vi "old version -- App - temperature sweep V0.vi"() -> ()   [LabVIEW 2010]
uses:
  state.ctl
  watch for sweep file.ctl
  save log.ctl
  save sweep table.ctl
  collect - input.ctl
  RUS/Controls/Sweep settings.ctl
  RUS/Controls/Lock-in DAQ settings.ctl
  File/Controls/Save data settings.ctl
  File/Controls/File formats.ctl
  ITC Panel.ctl
  collect.ctl
panel:
  out "Global stop indicator":bool
  in  "everything":T1(tab) caption="Tab Control"
  out "minutes/sweep":dbl=1.3333333333333333
  in  "save frequency in":bool=TRUE
  in  "Lock-in DAQ settings":T2={"Lockin mode"=enum."NI-DAQ", "DAQmx Device"="Dev2", "SR Lockin"="GPIB0::10::INSTR", "Clock Multiplier"=64, "Low-pass filter"=enum."No filtering", "Ranges and couplings "=[{"Range"=2.5, "Coupling"=10106}], "Samples per read"=10, "Record IF"=FALSE, "Auto-phase"=FALSE} {"Ranges and couplings"."Coupling" items=["default"=-1, "RSE"=10083, "NRSE"=10078, "Differential"=10106, "Pseudodifferential"=12529]}
  in  "Fast sweep settings":T3={"Update rate (Hz)"=250.0, "Start F, Hz"=900000.0, "Stop F"=1500000.0, "Number of points"=20000, "Amplitude"=2.1, "Init&amplitude"=TRUE, "IF"=1000.0, "Time constant"=0.003} {"IF" format="%#_6p"; "Amplitude" min=0.0 max=2.5; "Number of points" format="%.0p"; "Stop F" format="%#_6p"; "Start F, Hz" format="%#_6p"; "Update rate (Hz)" format="%0.2f"}
  in  "Stop RUS loop":bool
  in  "Save data settings":T4={"Save data"=TRUE, "Data Root Path"=path "C:/data/RUS/Experiment/ProbeTest/Probe10/saphire thin plate/sweep1", "File Prefix"="", "File Format"=enum."BINARY", "Save column names"=FALSE, "File Comments"="<Description of the current file>", "User/Prj"="<User Name/Project Description>"}
  in  "wait time between sweeps (min)":dbl
  in  "RUS loop":bool=TRUE
  in  "at end of every sweep":bool
  out "kHz/second":dbl=7.5
  in  "temperature boxes":T6={"LTC21 Address"="GPIB0::15::INSTR", "ITC503 Address"="GPIB0::24::INSTR", "ITC temperature"=159.22, "ITC set temperature"=159.23, "LTC temperature"=154.575, "heater"=11.7, "gas flow"=15.8, "P"=10.0, "D"=1.0, "I"=3.0, "ITC state"="X0A1C2S03H1L0\r", "nonzero temperature"=159.22}
  in  "Bypass error dialog":bool=TRUE
  out "Plot: heater/gas":cluster{dbl[], dbl[]}[](graph)
  out "heater slope, V/min":dbl=0.013240656024252648 format="%#.5f"
  out "heater average":dbl=11.680828906580725 format="%.3g"
  out "LTC T slope, K/min":dbl=0.38030539813461806 format="%#.5f"
  out "Plot: temperature":cluster{dbl[], dbl[]}[](graph)
  out "ITC Set T":dbl=159.23 format="%.3g"
  out "ITC Temperature":dbl=159.22 format="%.3g"
  out "LTC Temperature":dbl=154.575 format="%.3g"
  in  "show plot pallets":bool
  in  "set temperature to":bool
  in  "set temperature to":dbl=271.0
  in  "Tab: ITC controls":enum32{"Page 2"}(tab)
  in  "ITC panel":T7={"Locked"=FALSE, "Unlocked"=TRUE, "Remote"=FALSE, "Local"=TRUE, "in sweep"=TRUE, "start/stop sweep"=TRUE, "Sweep indicator"="IN sweep   2", "heater MANUAL"=FALSE, "heater AUTO"=TRUE, "ITC state"="X0A1C2S01H1L0\r", "gas MANUAL"=TRUE, "gas AUTO"=FALSE, "heater"=11.7, "gas flow %"=15.8} {"gas flow %" format="%.3g"; "heater" format="%.3g"}
  in  "Tab : Overheat":enum32{"Page 1"}(tab)
  in  "Over heat Temperature":dbl=350.0
  in  "Overheat protection":bool
  out "Overheat !!":bool
  in  "Tab : everything to zero":enum32{"Page 1", "Page 2"}(tab)
  in  "after (#min)":dbl=1600.0
  in  "everything to zero":bool
  in  "done":bool
  in  "to zero counter sec)":i32=132
  in  "to zero start (sec)":i32=-1
  in  "TAB: gas flow control":enum32{"Page 2"}(tab)
  in  "stop ramp up/down":bool
  in  "force ramp down now":bool
  in  "force ramp up now":bool
  in  "to":dbl=33.0
  in  "set gas flow":bool
  out "cycles between ramp up steps":i32=120
  out "ramp down in progress":bool
  out "ramp up in progress":bool
  in  "increase Gas % by":dbl=3.0
  out "(total # of ramp up steps)":i32=30
  in  "ramp up time (min)":dbl=60.0
  in  "ramp down time (min)":dbl=60.0
  in  "smallest ramp gas step":dbl=0.1
  out "(total # of ramp down steps)":i32=30
  out "ramp down steps so far":i32
  out "ramp up steps so far":i32
  out "Gas flow":dbl=15.8 format="%.2f"
  out "heater in range":bool=TRUE
  out "heater voltage":dbl=11.7 format="%.2f"
  in  "lower limit":dbl=3.0
  in  "upper limit":dbl=12.0
  in  "gas flow check interval (min)":dbl=11.0
  out "heater above":bool
  out "heater below":bool
  out "minutes since last check":i32=2
  in  "decrease Gas % by":dbl=3.0
  in  "Control Gas flow ?":bool=TRUE
  out "cycles between ramp down steps":i32=120
  in  "Tab: PID control":enum32{"Page 1"}(tab)
  in  "PID is":bool=TRUE
  out "D":dbl=1.0 format="%.2f"
  out "I":dbl=3.0 format="%.2f"
  out "P":dbl=10.0 format="%.2f"
  out "cycles since PID update":dbl=131.0 format="%.2f"
  in  "PID update every":i32=3600
  in  "PID table":dbl[][](array[numeric])=[[400.0, 10.0, 3.0, 1.0], [300.0, 10.0, 3.0, 1.0], [60.0, 10.0, 3.0, 1.0], [40.0, 10.0, 3.0, 1.0], [20.0, 30.0, 0.5, 0.2], [10.0, 40.0, 0.5, 0.2], [1.0, 50.0, 0.2, 0.2], [0.0, 50.0, 0.2, 0.2]]
  out "Uploading ...":bool
  in  "Tab : Upload Sweep table":enum32{"Page 1"}(tab)
  out "Sweep Rates , \nmin/K":dbl[][](array[numeric])=[[1.3761467889908257], [13.333333333333334], [8.0], [-0.0], [nan], [nan], [nan], [nan], [nan], [nan], [nan], [nan], [nan], [nan], [nan], [0.0]]
  out "current set \ntemperature":dbl=91.0
  in  "start \nset temperature":dbl=91.0
  in  "New Sweep Table":dbl[][](array[numeric])=[[200.0, 150.0, 0.0], [260.0, 800.0, 0.0], [310.0, 400.0, 0.0], [0.0, 0.0, 0.0], [0.0, 0.0, 0.0], [0.0, 0.0, 0.0], [0.0, 0.0, 0.0], [0.0, 0.0, 0.0], [0.0, 0.0, 0.0], [0.0, 0.0, 0.0], [0.0, 0.0, 0.0], [0.0, 0.0, 0.0], [0.0, 0.0, 0.0], [0.0, 0.0, 0.0], [0.0, 0.0, 0.0], [295.0, 0.0, 0.0]]
  in  "Read Sweep Table in the box":bool
  out "Sweep Table":dbl[][](array[numeric])=[[200.0, 150.0, 0.0], [260.0, 800.0, 0.0], [310.0, 400.0, 0.0], [0.0, 0.0, 0.0], [0.0, 0.0, 0.0], [0.0, 0.0, 0.0], [0.0, 0.0, 0.0], [0.0, 0.0, 0.0], [0.0, 0.0, 0.0], [0.0, 0.0, 0.0], [0.0, 0.0, 0.0], [0.0, 0.0, 0.0], [0.0, 0.0, 0.0], [0.0, 0.0, 0.0], [0.0, 0.0, 0.0], [295.0, 0.0, 0.0]]
  in  "upload new sweep table":bool
  out "Sweep Rates ,\nK/min":dbl[][](array[numeric])=[[0.7266666666666667], [0.075], [0.125], [-inf], [nan], [nan], [nan], [nan], [nan], [nan], [nan], [nan], [nan], [nan], [nan], [inf]]
  out "index":dbl[][](array[numeric])=[[0.0, 1200.0, 0.0], [1.0, 1200.0, 0.0], [2.0, 500.0, 0.0], [3.0, 1399.0, 0.0], [4.0, 10.0, 1399.0], [5.0, 10.0, 1399.0], [6.0, 0.0, 0.0], [7.0, 0.0, 0.0], [8.0, 0.0, 0.0], [9.0, 0.0, 0.0], [10.0, 0.0, 0.0], [11.0, 0.0, 0.0], [12.0, 0.0, 0.0], [13.0, 0.0, 0.0], [14.0, 0.0, 0.0], [15.0, 0.0, 0.0]]
  in  "New Sweep Sequence":dbl[][](array[numeric])=[[150.0, 1399.0, 0.0], [20.0, 1399.0, 0.0], [150.0, 1399.0, 0.0], [300.0, 1399.0, 0.0], [295.0, 10.0, 1399.0], [295.0, 10.0, 1399.0]]
  in  "upload new sweep sequence":bool
  in  "watch for sweep files in":T8={"file path"=path "C:/data/RUS/Experiment/ProbeTest/Probe10/saphire thin plate/sweep1", "Watch for sweep files?"=FALSE}
  out "milliseconds per cycle":u32=1000
  in  "Save sweep table":T9={"file path"=path "C:/data/RUS/Experiment/ProbeTest/probe9/LSCO_13/Sweep1", "Save sweep table?"=FALSE}
  in  "save log":T10={"file path"=path "C:/data/RUS/Experiment/ProbeTest/Probe10/saphire thin plate/sweep1", "Save log?"=TRUE, "every # of sec"=2}
  in  "bookkeeping":T11={"time(min)"=0.0, "T (ITC )"=159.22, "T (ITC, set)"=159.23, "heater"=11.7, "gas"=15.8, "T (ITC)  - T (ITC, set)"=-0.01654530309031088, "T (LTC)  - T (ITC, set)"=-4.661545303090321, "heater slope"=0.013240656024252648, "LTC slope"=0.38030539813461806, "hetaer running average"=11.680828906580725, "T (LTC)"=154.575, "T (LTC) running average"=154.57645899575306}
  out "heater":dbl=11.7 format="%.3g"
  out "gas flow %":dbl=15.8 format="%.3g"
  out "history length (min)":dbl=20.0
  out "cursor position":dbl=-1.0
  out "saving sweep table to":string
  out "saving log to":string="C:\\data\\RUS\\Experiment\\ProbeTest\\Probe10\\saphire thin plate\\sweep1\\Control_ITC_Log_120811.dat"
  out "history length (sec)":i32=1200
  out "minutes":dbl=2.183333333333333
  out "seconds":i32=131
  out "sweep files in the folder":i32=-1
  in  "error in":errorcluster
  out "error out":errorcluster
  out "log line":string="time=Dec08,2011__10:59:36\tLTC=153.75300\tITC=158.40000\t ITC_set=158.42000\t\t filename=158.40000K_900_1500_120811.dat\t"
  out "writing log to":string="C:\\data\\RUS\\Experiment\\ProbeTest\\Probe10\\saphire thin plate\\sweep1\\Stability_120811.dat"
  in  "event loop":bool
  # "cycles"
  # "Temp (K)                  P                          I                         D"
  # "the paths are copied from \"data root path\" in the first page"
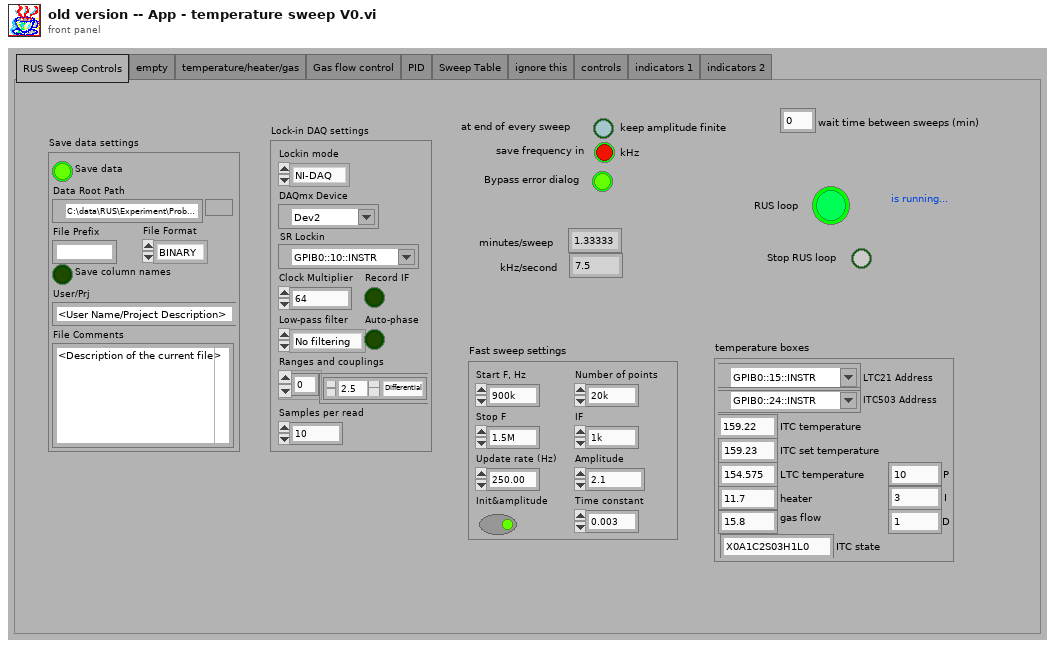
[diagram p1: front panel]
types:
  T1 = enum32{"RUS Sweep Controls", "empty", "temperature/heater/gas", "Gas flow control", "PID", "Sweep Table", "ignore this", "controls", "indicators 1", "indicators 2"}
  T2 = typedef "Lock-in DAQ settings.ctl" = cluster{"Lockin mode":enum16{"SRS", "NI-DAQ"}, "DAQmx Device":tag, "SR Lockin":refnum<visa-resource-name>, "Clock Multiplier":i32, "Low-pass filter":enum16{"No filtering", "Butterworth", "Bessel"}, "Ranges and couplings ":cluster{"Range":dbl, "Coupling":i32}[], "Samples per read":i32, "Record IF":bool, "Auto-phase":bool}
  T3 = typedef "Sweep settings.ctl" = cluster{"Update rate (Hz)":dbl, "Start F, Hz":dbl, "Stop F":dbl, "Number of points":i32, "Amplitude":dbl, "Init&amplitude":bool, "IF":dbl, "Time constant":dbl}
  T4 = typedef "Save data settings.ctl" = cluster{"Save data":bool, "Data Root Path":path, "File Prefix":string, "File Format":T5, "Save column names":bool, "File Comments":string, "User/Prj":string}
  T5 = typedef "File formats.ctl" = enum16{"TDMS", "ASCII", "BINARY"}
  T6 = typedef "state.ctl" = cluster{"LTC21 Address":refnum<visa-resource-name>, "ITC503 Address":refnum<visa-resource-name>, "ITC temperature":dbl, "ITC set temperature":dbl, "LTC temperature":dbl, "heater":dbl, "gas flow":dbl, "P":dbl, "D":dbl, "I":dbl, "ITC state":string, "nonzero temperature":dbl}
  T7 = typedef "ITC Panel.ctl" = cluster{"Locked":bool, "Unlocked":bool, "Remote":bool, "Local":bool, "in sweep":bool, "start/stop sweep":bool, "Sweep indicator":string, "heater MANUAL":bool, "heater AUTO":bool, "ITC state":string, "gas MANUAL":bool, "gas AUTO":bool, "heater":dbl, "gas flow %":dbl}
  T8 = typedef "watch for sweep file.ctl" = cluster{"file path":path, "Watch for sweep files?":bool}
  T9 = typedef "save sweep table.ctl" = cluster{"file path":path, "Save sweep table?":bool}
  T10 = typedef "save log.ctl" = cluster{"file path":path, "Save log?":bool, "every # of sec":i32}
  T11 = typedef "collect - input.ctl" = cluster{"time(min)":dbl, "T (ITC )":dbl, "T (ITC, set)":dbl, "heater":dbl, "gas":dbl, "T (ITC)  - T (ITC, set)":dbl, "T (LTC)  - T (ITC, set)":dbl, "heater slope":dbl, "LTC slope":dbl, "hetaer running average":dbl, "T (LTC)":dbl, "T (LTC) running average":dbl}
  T12 = typedef "collect.ctl" = cluster{"time(min)":dbl[], "T (ITC )":dbl[], "T (ITC, set)":dbl[], "T (LTC)":dbl[], "heater":dbl[], "gas":dbl[], "T (ITC)  - T (ITC, set)":dbl[], "T (LTC)  - T (ITC, set)":dbl[], "heater slope":dbl[], "LTC slope":dbl[], "hetaer running average":dbl[], "T (LTC) running average":dbl[]}
  T13 = enum8{"Enabled", "Disabled", "Disabled and Grayed Out"}
  T14 = enum32{"Page Enabled", "Page Disabled", "Page Disabled & Grayed"}
  T15 = cluster{"time(min)":dbl[], "T (ITC)  - T (ITC, set)":dbl[]}
  T16 = cluster{"time(min)":dbl[], "T (LTC)  - T (ITC, set)":dbl[]}
  T17 = cluster{"time(min)":dbl[], "heater slope":dbl[]}[]
  T18 = enum16{"parse", "start sweep", "stop sweep", "heater auto", "heater manual", "set heater"}
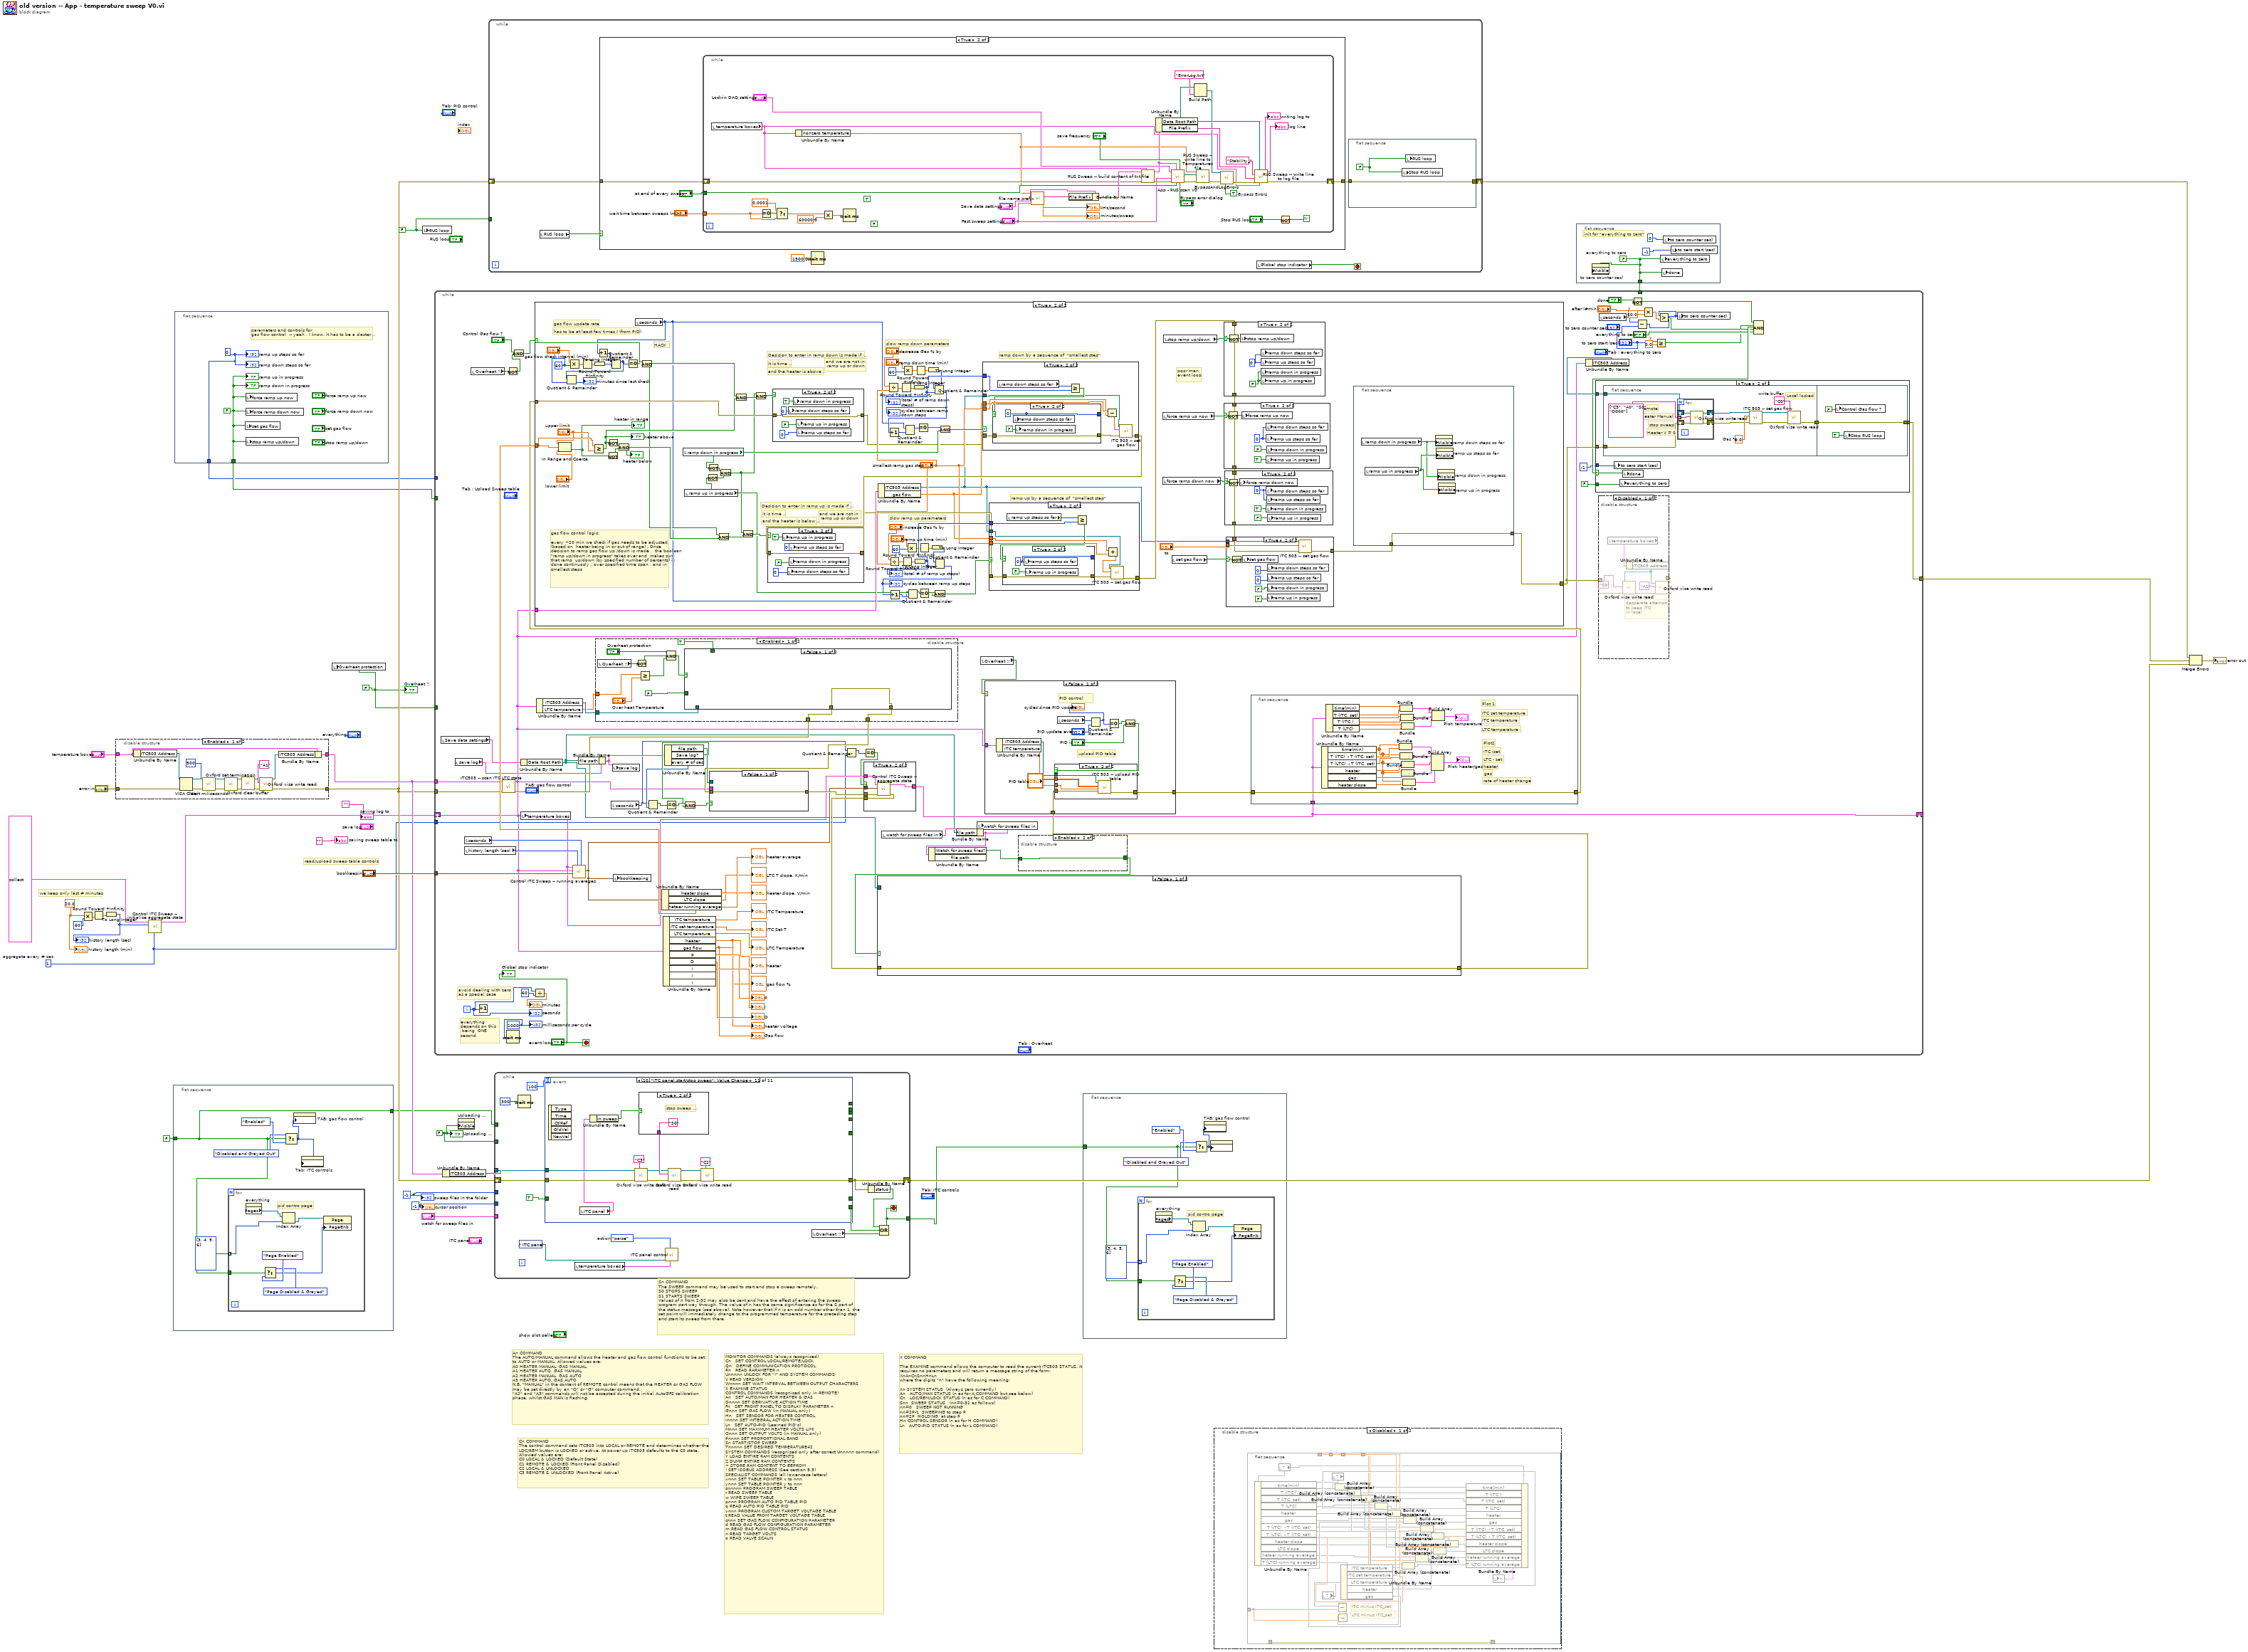
[diagram p0: block diagram]
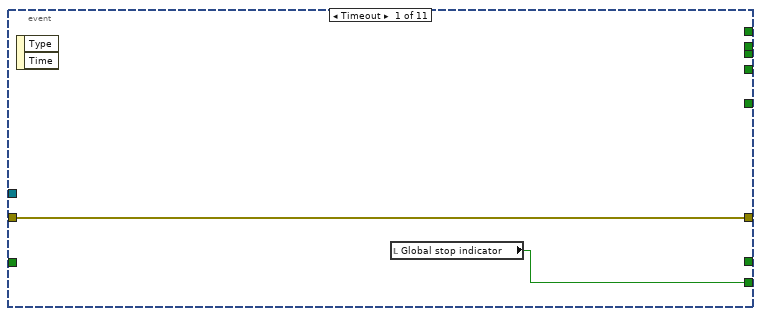
[diagram p3: hidden frame]
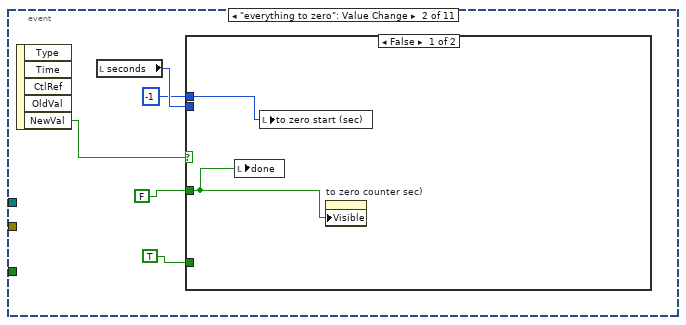
[diagram p4: hidden frame]
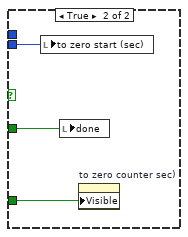
[diagram p5: hidden frame]
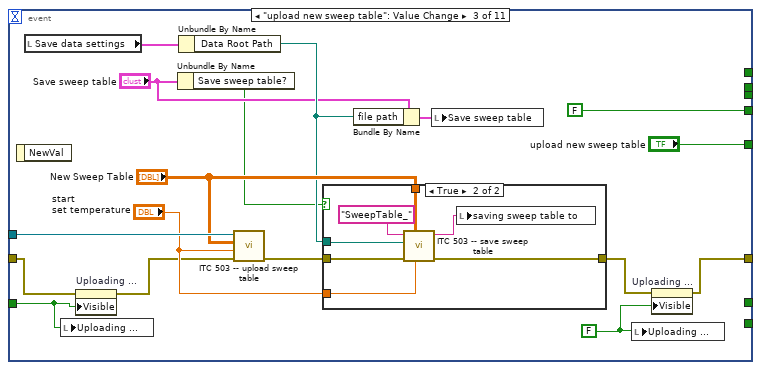
[diagram p6: hidden frame]
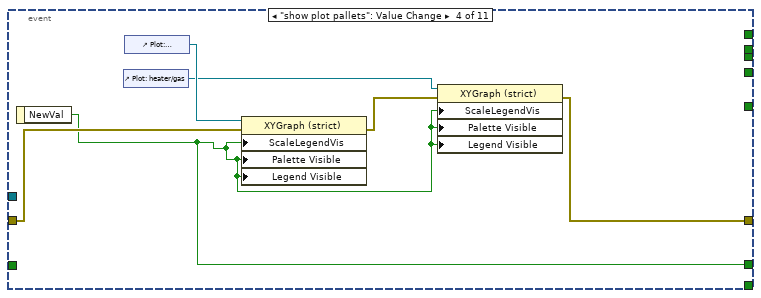
[diagram p8: hidden frame]
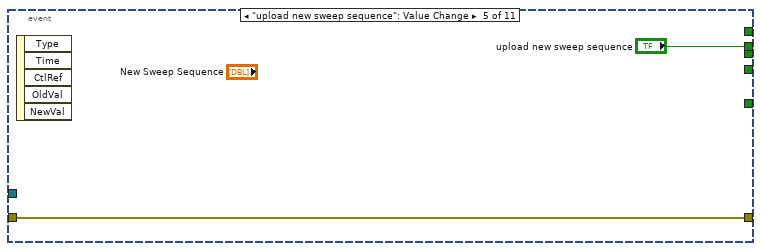
[diagram p9: hidden frame]
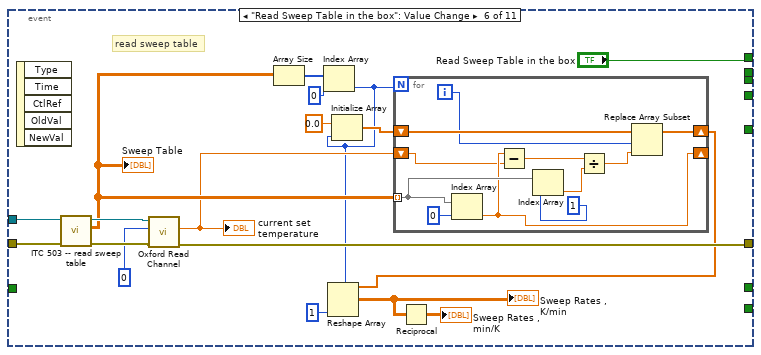
[diagram p10: hidden frame]
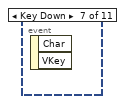
[diagram p11: hidden frame]
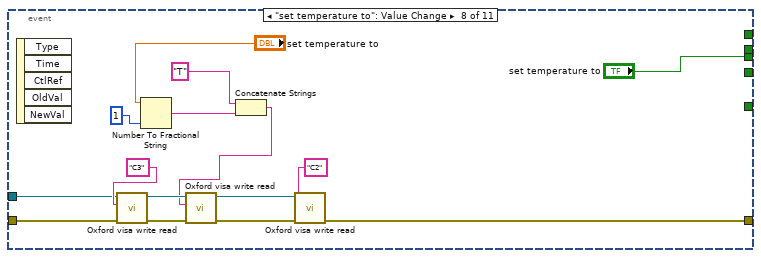
[diagram p12: hidden frame]
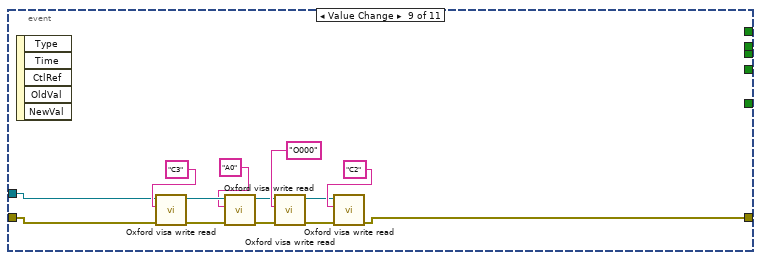
[diagram p13: hidden frame]
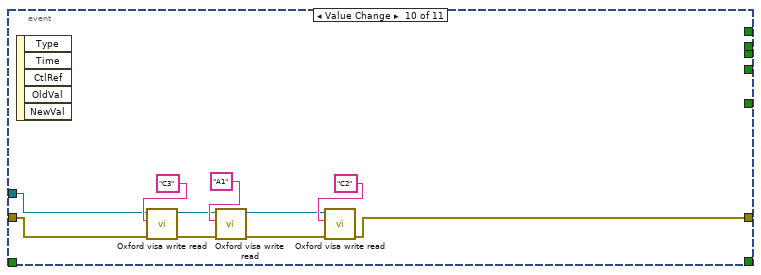
[diagram p14: hidden frame]
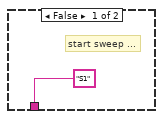
[diagram p15: hidden frame]
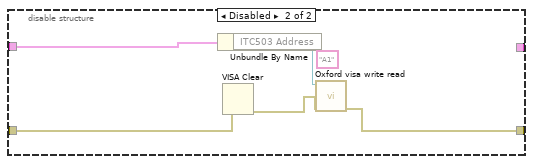
[diagram p16: hidden frame]
diagram:
  w4 = u32 1  # aggregate every # sec
  w12 = FALSE
  w11 = FALSE ("Start RUS Sweep loop")
  w14 = -1
  w29 = 20.0 ("standard deviation")
  w15 = -1 ("sweep files in the folder")
  w7 = FALSE
  # "Cn COMMAND\nThe control command sets ITC503 into LOCAL or REMOTE and determines whether the\nLOC/REM button is LOCKED or active. At power up ITC503 defaults to the C0 state.\nAllowed values are:\nC0 LOCAL & LOCKED (Default State)\nC1 REMOTE & LOCKED (Front Panel Disabled)\nC2 LOCAL & UNLOCKED\nC3 REMOTE & UNLOCKED (Front Panel Active)"
  # "An COMMAND\nThe AUTO/MANUAL command allows the heater and gas flow control functions to be set\nto AUTO or MANUAL. Allowed values are:\nA0 HEATER MANUAL, GAS MANUAL\nA1 HEATER AUTO, GAS MANUAL\nA2 HEATER MANUAL, GAS AUTO\nA3 HEATER AUTO, GAS AUTO\nN.B. \"MANUAL\" in the context of REMOTE control means that the HEATER or GAS FLOW\nmay be set directly by an \"O\" or \"G\" computer command.\n\"A2\" and \"A3\" commands will not be accepted during the initial AutoGFS calibration\nphase, whilst GAS MAN is flashing."
  # "MONITOR COMMANDS (always recognised)\nCn   SET CONTROL LOCAL/REMOTE/LOCK\nQn   DEFINE COMMUNICATION PROTOCOL\nRn   READ PARAMETER n\nUnnnnn UNLOCK FOR \"!\" AND SYSTEM COMMANDS\nV READ VERSION\nWnnnn SET WAIT INTERVAL BETWEEN OUTPUT CHARACTERS\nX EXAMINE STATUS\nCONTROL COMMANDS (recognised only in REMOTE)\nAn   SET AUTO/MAN FOR HEATER & GAS\nDnnnn SET DERIVATIVE ACTION TIME\nFn   SET FRONT PANEL TO DISPLAY PARAMETER n\nGnnn SET GAS FLOW (in MANUAL only)\nHn   SET SENSOR FOR HEATER CONTROL\nInnnn SET INTEGRAL ACTION TIME\nLn   SET AUTO-PID (Learned PID's)\nMnnn SET MAXIMUM HEATER VOLTS LIMI\nOnnn SET OUTPUT VOLTS (in MANUAL only)\nPnnnn SET PROPORTIONAL BAND\nSn START/STOP SWEEP\nTnnnnn SET DESIRED TEMPERATURE42\nSYSTEM COMMANDS (recognised only after correct Unnnnn command)\nY LOAD ENTIRE RAM CONTENTS\nZ DUMP ENTIRE RAM CONTENTS\n~ STORE RAM CONTENT TO EEPROM\n! SET ISOBUS ADDRESS (See section 8.5)\nSPECIALIST COMMANDS (all lower-case letters)\nxnnn SET TABLE POINTER x to nnn\nynnn SET TABLE POINTER y to nnn\nsnnnnn PROGRAM SWEEP TABLE\nr READ SWEEP TABLE\nw WIPE SWEEP TABLE\npnnn PROGRAM AUTO PID TABLE PID\nq READ AUTO PID TABLE PID\nvnnn PROGRAM CUSTOM TARGET VOLTAGE TABLE\nt READ VALUE FROM TARGET VOLTAGE TABLE\ncnnn SET GAS FLOW CONFIGURATION PARAMETER\nd READ GAS FLOW CONFIGURATION PARAMETER\nm READ GAS FLOW CONTROL STATUS\nn READ TARGET VOLTS\no READ VALVE SCALIN"
  # "X COMMAND\n\nThe EXAMINE command allows the computer to read the current ITC503 STATUS. It\nrequires no parameters and will return a message string of the form:\nXnAnCnSnnHnLn\nwhere the digits \"n\" have the following meaning:\n\nXn SYSTEM STATUS  (Always zero currently)\nAn   AUTO/MAN STATUS (n as for A COMMAND but see below)\nCn   LOC/REM/LOCK STATUS (n as for C COMMAND)\nSnn  SWEEP STATUS   (nn=0-32 as follows)\nnn=0   SWEEP NOT RUNNING\nnn=2P-1  SWEEPING to step P\nnn=2P  HOLDING  at step P\nHn CONTROL SENSOR (n as for H COMMAND)\nLn   AUTO-PID STATUS (n as for L COMMAND)"
  # "Sn COMMAND\nThe SWEEP command may be used to start and stop a sweep remotely.\nS0 STOPS SWEEP\nS1 STARTS SWEEP\nValues of n from 2-32 may also be sent and have the effect of entering the sweep\nprogram part way through. The value of n has the same significance as for the S part of\nthe status message (see above). Note however that if n is an odd number other than 1, the\nset point will immediately change to the programmed temperature for the preceding step\nand start its sweep from there."
  # "read/upload sweep table controls"
  # "we keep only last # minutes"
  n1 = Multiply(x=w29, y=60) -> (x*y=w32:dbl)
  n2 = Round Toward +Infinity(x=w32) -> (ceil(x): smallest int >= x=w31:dbl)
  n3 = To Long Integer(number=w31) -> (32bit integer=w21:i32)
  "history length (sec)" <- w21
  n4 = disable-structure shown="Enabled" {
    disable-tunnel: "error in" -> [w45 w53]
    disable-tunnel: [w46 w48] -> w17
    disable-tunnel: "temperature boxes" -> [w42 w51]
    disable-tunnel: [w43 _] -> w20
    frame Enabled {
      n5 = Unbundle By Name(w42) -> ("ITC503 Address"=w41:refnum<visa-resource-name>)
      n6 = VISA Clear(VISA resource name=w41, error in (no error)=w45) -> (VISA resource name out=w47:refnum<visa-resource-name>, error out=w35:errorcluster)
      n7 = call "Wait miliseconds.vi"("error in (no error)"=w35, "milliseconds to wait"=u32 500) -> ("error out"=w34:errorcluster)  [unwired: 8 in, 1 out]
      n8 = call "Oxford set termination.vi"("error in (no error)"=w34, "VISA resource name"=w47) -> ("error out"=w40:errorcluster, "VISA resource name out"=w38:refnum<visa-resource-name>)  [unwired: 8 in]
      n9 = call "Oxford clear buffer.vi"("error in (no error)"=w40, "VISA resource name"=w38) -> ("error out"=w39:errorcluster, "VISA resource name out"=w37:refnum<visa-resource-name>)  [unwired: 6 in, 2 out]
      n10 = call "Oxford visa write read.vi"("error in (no error)"=w39, "write buffer"="A1" ("Command"), "VISA resource name"=w37) -> ("error out"=w46:errorcluster, "VISA resource name out"=w36:refnum<visa-resource-name>)  [unwired: 6 in, 1 out]
      n11 = Bundle By Name(cluster=w42, "ITC503 Address"=w36) -> (w43:T6)
    }
    frame Disabled {
      (unwired) "A1" ("Command")
      n12 = Unbundle By Name(w51) -> ("ITC503 Address"=w50:refnum<visa-resource-name>)
      n13 = VISA Clear(error in (no error)=w53) -> (VISA resource name=w52:refnum<visa-resource-name>, error out=w49:errorcluster)  [unwired: 1 out]
      n14 = call "Oxford visa write read.vi"("error in (no error)"=w49, "VISA resource name"=w50) -> ("error out"=w48:errorcluster)  [unwired: 7 in, 2 out]
    }
  }
  n15 = call "Control ITC Sweep -- initialize aggregate state.vi"("time step"=w4, "length"=w21, "more state -- aggregate in"=T12 {"time(min)"=array[7200 elements], "T (ITC )"=array[7200 elements], "T (ITC, set)"=array[7200 elements], "T (LTC)"=array[7200 elements], "heater"=array[7200 elements], "gas"=array[7200 elements], "T (ITC)  - T (ITC, set)"=array[7200 elements], "T (LTC)  - T (ITC, set)"=array[7200 elements], "heater slope"=array[7200 elements], "LTC slope"=array[7200 elements], "hetaer running average"=array[7200 elements], "T (LTC) running average"=array[7200 elements]} ("thermometer snapshot -- aggregate")) -> ("more state -- aggregate out"=w6:T12)  [unwired: 7 in, 1 out]
  n16 = flat-sequence {
    tunnel: FALSE -> [w54]
    tunnel: [w54] -> w8
    frame #0 {
      n17 = for {
        tunnel: w54 -> [w63]
        tunnel: i32[] [3, 4, 5, 6] -> [w59] mode=indexing
        # "pid contro page"
        n18 = property on="everything" class="TabCtl (strict)"() -> ("Pages"=w65:refnum<vi>[])  [unwired: 2 in, 2 out]
        n19 = Select(t=T14."Page Disabled & Grayed" ("Page Enabled State"), s=w63, f=T14."Page Enabled" ("Page Enabled State")) -> (s? t:f=w60:T14)
        n20 = Index Array(array=w65, index=w59) -> (element=w64:refnum<vi>)
        n21 = property on="Property Node" class="Page"(reference=w64, "PageEnb"=w60) -> ()  [unwired: 1 in, 2 out]
      }
      n22 = Select(t=T13."Disabled and Grayed Out" ("Disabled"), s=w54, f=T13."Enabled" ("Disabled")) -> (s? t:f=w56:T13)
      n23 = property on="TAB: gas flow control" class="TabCtl (strict)"("DisabledEnum"=w56) -> ()  [unwired: 2 in, 2 out]
      n24 = property on="Tab: ITC controls" class="TabCtl (strict)"("DisabledEnum"=w56) -> ()  [unwired: 2 in, 2 out]
    }
  }
  n25 = flat-sequence {
    tunnel: [w67] -> w3
    tunnel: [w66] -> w2
    frame #0 {
      w67 = FALSE ("set gas flow manually")
      w66 = 0 ("ramp up counter")
      # "parameters and controls for \ngas flow control  -- yeah , I know, it has to be a claster .."
      n26 = local write "set gas flow"(w67) -> ()
      n27 = local write "force ramp up now"(w67) -> ()
      n28 = local write "force ramp down now"(w67) -> ()
      n29 = local write "stop ramp up/down"(w67) -> ()
      "ramp up in progress" <- w67
      "ramp down in progress" <- w67
      "ramp up steps so far" <- w66
      "ramp down steps so far" <- w66
    }
  }
  n30 = local write "Overheat protection"(w12) -> ()
  n31 = local write "RUS loop"(w11) -> ()
  n32 = while {
    tunnel: w17 -> [w118]
    tunnel: [w83] -> w23
    tunnel: w20 -> [w119]
    tunnel: "bookkeeping" -> [w116]
    tunnel: w12 -> [_]
    shift-right: [w91] -> _
    shift-left: w6 -> [w92]
    tunnel: w4 -> [w88]
    tunnel: w3 -> [_]
    tunnel: w2 -> [_]
    tunnel: w1 -> [_]
    i -> [w132]
    stop <- "event loop" stop-if-true
    w75 = 0.0  # y
    w73 = 60.0  # y
    w142 = u32 1000 ("milliseconds per cycle")
    # "everything depends on this\n being  ONE second"
    # "avoid dealing with zero \nas a special case"
    n33 = local read "Save data settings"() -> (w98:T4)
    n34 = local read "save log"() -> (w97:T10)
    n35 = local read "seconds"() -> (w115:i32)
    n36 = local read "history length (sec)"() -> (w114:i32)
    n37 = local read "Overheat !!"() -> (w102:bool)
    n38 = Increment(x=w132) -> ()  [unwired: 1 out]
    n39 = call "ITC503 -- scan ITC LTC state.vi"("error in"=w118, "state IN"=w119) -> ("error out"=w107:errorcluster, "state OUT"=w82:T6)  [unwired: 8 in]
    n40 = Wait (ms)(milliseconds to wait=w142) -> ()  [unwired: 1 out]
    n41 = Not(x=w102) -> (.not. x?=w101:bool)
    n42 = And(x="Control Gas flow ?", y=w101) -> (x .and. y?=w99:bool)
    n43 = Unbundle By Name(w98) -> ("Data Root Path"=w94:path)
    n44 = local write "temperature boxes"(w82) -> ()
    n45 = Divide(x=w132, y=60) -> (x/y=→"minutes":dbl)
    n46 = Unbundle By Name(w82) -> ("ITC503 Address"=w105:refnum<visa-resource-name>, "LTC temperature"=w104:dbl)
    n47 = call "Control ITC Sweep -- running averages.vi"("seconds"=w115, "history length (sec)"=w114, "more state"=w116, "thermometer reading"=w82, "more state -- aggregate"=w92) -> ("more state out"=w111:T11)  [unwired: 6 in]
    n48 = Bundle By Name(cluster=w97, "file path"=w94) -> (w96:T10)
    n49 = disable-structure shown="Enabled" {
      disable-tunnel: w104 -> [w368 _]
      disable-tunnel: w105 -> [w367 _]
      disable-tunnel: w107 -> [w366 w383]
      disable-tunnel: [w365 w383] -> w106
      frame Enabled {
        n50 = local read "Overheat !!"() -> (w362:bool)
        n51 = Not(x=w362) -> (.not. x?=w361:bool)
        n52 = Greater Or Equal?(x=w368, y="Over heat Temperature") -> (x >= y?=w363:bool)
        n53 = Compound Arithmetic op=AND("Overheat protection", w361, w363) -> (w364:bool)
        n54 = case shown="False" w364 {
          tunnel: w367 -> [_ w378]
          tunnel: FALSE ("Control Gas flow ?") -> [_ w375]
          tunnel: TRUE ("Boolean") -> [_ w376]
          tunnel: w366 -> [w372 w374]
          tunnel: [w372 w373] -> w365
          frame False {
          }
          frame True {
            # "Local locked"
            # "Heater V = 0"
            # "Heater Manual"
            # "Remote"
            n55 = local write "Control Gas flow ?"(w375) -> ()
            n56 = local write "Overheat !!"(w376) -> ()
            n57 = for {
              tunnel: w378 -> [w382]
              tunnel: string[] ["C3", "A0", "O0", "C0"] -> [w381] mode=indexing
              tunnel: w374 -> [w380]
              tunnel: [w379] -> w373
              n58 = call "Oxford visa write read.vi"("error in (no error)"=w380, "write buffer"=w381, "VISA resource name"=w382) -> ("error out"=w379:errorcluster)  [unwired: 6 in, 2 out]
            }
          }
        }
      }
      frame Disabled {
      }
    }
    n59 = local read "seconds"() -> (w89:i32)
    n60 = local write "save log"(w96) -> ()
    n61 = local write "bookkeeping"(w111) -> ()
    n62 = Unbundle By Name(w111) -> ("heater slope"=→"heater slope, V/min":dbl, "LTC slope"=→"LTC T slope, K/min":dbl, "hetaer running average"=w128:dbl)
    "heater average" <- w128
    n63 = case shown="True" w99 {
      selector: w99 -> [_ w267]
      tunnel: w128 -> [_ w271]
      tunnel: [w195 w270] -> w84
      tunnel: w109 -> [w195 w269]
      tunnel: w82 -> [_ w268]
      frame False {
      }
      frame True {
        w201 = 60 ("y")
        # "ramp down by a sequence of  \"smallest step\""
        # "ramp up by a sequence of  \"smallest step\""
        # "HACK"
        # "poor man \nevent loop"
        # "and we are not in\n ramp up or down"
        # "Desicion to enter in ramp up is made if ..."
        # "and the heater is below .."
        # "it is time .."
        # "and we are not in\n ramp up or down"
        # "Desicion to enter in ramp down is made if ..."
        # "and the heater is above .."
        # "it is time .."
        # "slow ramp down parameters"
        # "slow ramp up parameters"
        # "gas flow control logic: \n\nevery ~20 min we check if gas needs to be adjusted  (based on  heater being in or out of range) . Once  decision to ramp gas flow up /down is made ,  the boolean \"ramp up/down in progress\" takes over and  makes sure that ramp  up/down (by specified number of percents) is done continuosly , over specified time span , and in smallest steps"
        # "has to be at least few times I (from PID)"
        # "gas flow update rate"
        n64 = In Range and Coerce(upper limit="upper limit", x=w271, lower limit="lower limit") -> (In Range?=w262:bool)  [unwired: 1 out]
        "heater in range" <- w262
        n65 = Multiply(x="gas flow check interval (min)", y=w201) -> (x*y=w221:dbl)
        n66 = Round Toward +Infinity(x=w221) -> (ceil(x): smallest int >= x=w220:dbl)
        n67 = Greater Or Equal?(x=w271, y="upper limit") -> (x >= y?=w260:bool)
        "heater above" <- w260
        n68 = To Long Integer(number=w220) -> (32bit integer=w218:i32)
        n69 = Not(x=w262) -> (.not. x?=w264:bool)
        n70 = Not(x=w260) -> (.not. x?=w263:bool)
        n71 = And(x=w263, y=w264) -> (x .and. y?=w254:bool)
        "heater below" <- w254
        n72 = local read "seconds"() -> (w199:i32)
        n73 = Increment(x=w199) -> (x+1=w198:i32)
        n74 = Quotient & Remainder(x=w198, y=w218) -> (x-y*floor(x/y)=w202:i32)  [unwired: 1 out]
        n75 = Quotient & Remainder(x=w202, y=w201) -> (floor(x/y)=→"minutes since last check":i32)  [unwired: 1 out]
        n76 = Equal To 0?(x=w202) -> (x = 0?=w261:bool)
        n77 = And(x=w267, y=w261) -> (x .and. y?=w244:bool)
        n78 = local read "ramp down in progress"() -> (w257:bool)
        n79 = local read "ramp up in progress"() -> (w241:bool)
        n80 = Not(x=w241) -> (.not. x?=w248:bool)
        n81 = Not(x=w257) -> (.not. x?=w249:bool)
        n82 = And(x=w244, y=w254) -> (x .and. y?=w255:bool)
        n83 = And(x=w249, y=w248) -> (x .and. y?=w246:bool)
        n84 = And(x=w244, y=w260) -> (x .and. y?=w259:bool)
        n85 = And(x=w246, y=w255) -> (x .and. y?=w245:bool)
        n86 = And(x=w246, y=w259) -> (x .and. y?=w247:bool)
        n87 = case shown="True" w247 {
          tunnel: [w329 w333] -> w205
          tunnel: w269 -> [w329 w333]
          frame False {
          }
          frame True {
            n88 = local write "ramp down steps so far"(0 ("ramp down counter")) -> ()
            n89 = local write "ramp down in progress"(TRUE ("ramp down in progress")) -> ()
            n90 = local write "ramp up in progress"(FALSE ("ramp down in progress")) -> ()
            n91 = local write "ramp up steps so far"(0 ("ramp down counter")) -> ()
          }
        }
        n92 = Unbundle By Name(w268) -> ("ITC503 Address"=w196:refnum<visa-resource-name>, "gas flow"=w207:dbl)
        n93 = Divide(x="decrease Gas % by", y="smallest ramp gas step") -> (x/y=w231:dbl)
        n94 = Divide(x="increase Gas % by", y="smallest ramp gas step") -> (x/y=w236:dbl)
        n95 = Round Toward +Infinity(x=w231) -> (ceil(x): smallest int >= x=w230:dbl)
        n96 = Round Toward +Infinity(x=w236) -> (ceil(x): smallest int >= x=w234:dbl)
        n97 = Multiply(x="ramp down time (min)", y=60) -> (x*y=w217:dbl)
        n98 = Multiply(x="ramp up time (min)", y=60) -> (x*y=w212:dbl)
        n99 = To Long Integer(number=w230) -> (32bit integer=w227:i32)
        "(total # of ramp down steps)" <- w227
        n100 = To Long Integer(number=w234) -> (32bit integer=w233:i32)
        "(total # of ramp up steps)" <- w233
        n101 = Round Toward +Infinity(x=w217) -> (ceil(x): smallest int >= x=w216:dbl)
        n102 = Round Toward +Infinity(x=w212) -> (ceil(x): smallest int >= x=w211:dbl)
        n103 = To Long Integer(number=w216) -> (32bit integer=w213:i32)
        n104 = To Long Integer(number=w211) -> (32bit integer=w209:i32)
        n105 = Quotient & Remainder(x=w213, y=w227) -> (floor(x/y)=w226:i32)  [unwired: 1 out]
        "cycles between ramp down steps" <- w226
        n106 = Increment(x=w226) -> (x+1=w240:i32)
        n107 = Quotient & Remainder(x=w199, y=w240) -> (x-y*floor(x/y)=w258:i32)  [unwired: 1 out]
        n108 = Equal To 0?(x=w258) -> (x = 0?=w239:bool)
        n109 = Quotient & Remainder(x=w209, y=w233) -> (floor(x/y)=w232:i32)  [unwired: 1 out]
        "cycles between ramp up steps" <- w232
        n110 = Increment(x=w232) -> (x+1=w237:i32)
        n111 = Quotient & Remainder(x=w199, y=w237) -> (x-y*floor(x/y)=w251:i32)  [unwired: 1 out]
        n112 = Equal To 0?(x=w251) -> (x = 0?=w238:bool)
        n113 = And(x=w241, y=w238) -> (x .and. y?=w250:bool)
        n114 = And(x=w239, y=w257) -> (x .and. y?=w256:bool)
        n115 = case shown="True" w256 {
          tunnel: w207 -> [_ w345]
          tunnel: w196 -> [_ w339]
          tunnel: [w335 w338] -> w253
          tunnel: "smallest ramp gas step" -> [_ w344]
          tunnel: w227 -> [_ w341]
          tunnel: w205 -> [w335 w336]
          frame False {
          }
          frame True {
            n116 = local read "ramp down steps so far"() -> (w343:i32)
            n117 = Greater Or Equal?(x=w343, y=w341) -> (x >= y?=w342:bool)
            n118 = case shown="True" w342 {
              tunnel: [w346 w351] -> w337
              tunnel: w336 -> [w346 w351]
              tunnel: [w347 w350] -> _
              frame False {
                n119 = local read "ramp down steps so far"() -> (w347:i32)
                n120 = Increment(x=w347) -> (x+1=w348:i32)
                n121 = local write "ramp down steps so far"(w348) -> ()
              }
              frame True {
                w350 = 0 ("ramp down counter")
                n122 = local write "ramp down steps so far"(w350) -> ()
                n123 = local write "ramp down in progress"(FALSE ("ramp down in progress")) -> ()
              }
            }
            n124 = Subtract(x=w345, y=w344) -> (x-y=w340:dbl)
            n125 = call "ITC 503 -- set gas flow.vi"("error in"=w337, "Gas %"=w340, "ITC503 Address"=w339) -> ("error out"=w338:errorcluster)  [unwired: 7 in, 1 out]
          }
        }
        n126 = case shown="True" w245 {
          tunnel: w253 -> [w323 w327]
          tunnel: [w323 w327] -> w252
          frame False {
          }
          frame True {
            n127 = local write "ramp up in progress"(TRUE ("ramp up in progress")) -> ()
            n128 = local write "ramp down steps so far"(0 ("ramp down counter")) -> ()
            n129 = local write "ramp down in progress"(FALSE ("ramp down in progress")) -> ()
            n130 = local write "ramp up steps so far"(0 ("ramp up counter")) -> ()
          }
        }
        n131 = case shown="True" w250 {
          tunnel: w207 -> [_ w316]
          tunnel: w196 -> [_ w307]
          tunnel: w252 -> [w306 w314]
          tunnel: [w306 w310] -> w204
          tunnel: "smallest ramp gas step" -> [_ w315]
          tunnel: w233 -> [_ w311]
          frame False {
            # "heater above ..."
          }
          frame True {
            n132 = local read "ramp up steps so far"() -> (w313:i32)
            n133 = Greater Or Equal?(x=w313, y=w311) -> (x >= y?=w312:bool)
            n134 = case shown="True" w312 {
              tunnel: [w317 w322] -> w309
              tunnel: w314 -> [w317 w322]
              tunnel: [w318 w321] -> _
              frame False {
                n135 = local read "ramp up steps so far"() -> (w318:i32)
                n136 = Increment(x=w318) -> (x+1=w319:i32)
                n137 = local write "ramp up steps so far"(w319) -> ()
              }
              frame True {
                w321 = 0 ("ramp down counter")
                n138 = local write "ramp up steps so far"(w321) -> ()
                n139 = local write "ramp up in progress"(FALSE ("ramp down in progress")) -> ()
              }
            }
            n140 = Add(x=w316, y=w315) -> (x+y=w308:dbl)
            n141 = call "ITC 503 -- set gas flow.vi"("error in"=w309, "Gas %"=w308, "ITC503 Address"=w307) -> ("error out"=w310:errorcluster)  [unwired: 7 in, 1 out]
          }
        }
        n142 = local read "force ramp up now"() -> (w225:bool)
        n143 = local read "force ramp down now"() -> (w224:bool)
        n144 = local read "stop ramp up/down"() -> (w206:bool)
        n145 = local read "set gas flow"() -> (w242:bool)
        n146 = case shown="True" w206 {
          selector: w206 -> [_ w277]
          tunnel: w204 -> [w275 w279]
          tunnel: [w275 w279] -> w203
          frame False {
          }
          frame True {
            w280 = 0
            w278 = FALSE
            n147 = Not(x=w277) -> (.not. x?=w276:bool)
            n148 = local write "stop ramp up/down"(w276) -> ()
            n149 = local write "ramp down steps so far"(w280) -> ()
            n150 = local write "ramp up steps so far"(w280) -> ()
            n151 = local write "ramp down in progress"(w278) -> ()
            n152 = local write "ramp up in progress"(w278) -> ()
          }
        }
        n153 = case shown="True" w225 {
          selector: w225 -> [_ w291]
          tunnel: [w288 w294] -> w223
          tunnel: w203 -> [w288 w294]
          frame False {
          }
          frame True {
            w289 = 0 ("ramp up counter")
            n154 = Not(x=w291) -> (.not. x?=w292:bool)
            n155 = local write "force ramp up now"(w292) -> ()
            n156 = local write "ramp down steps so far"(w289) -> ()
            n157 = local write "ramp up steps so far"(w289) -> ()
            n158 = local write "ramp up in progress"(TRUE ("ramp up in progress")) -> ()
            n159 = local write "ramp down in progress"(FALSE) -> ()
          }
        }
        n160 = case shown="True" w224 {
          selector: w224 -> [_ w285]
          tunnel: w223 -> [w281 w287]
          tunnel: [w281 w287] -> w222
          frame False {
          }
          frame True {
            w283 = 0 ("ramp down counter")
            n161 = Not(x=w285) -> (.not. x?=w284:bool)
            n162 = local write "force ramp down now"(w284) -> ()
            n163 = local write "ramp down steps so far"(w283) -> ()
            n164 = local write "ramp down in progress"(TRUE ("ramp down in progress")) -> ()
            n165 = local write "ramp up steps so far"(w283) -> ()
            n166 = local write "ramp up in progress"(FALSE) -> ()
          }
        }
        n167 = case shown="True" w242 {
          selector: w242 -> [_ w297]
          tunnel: "to" -> [_ w302]
          tunnel: w222 -> [w295 w301]
          tunnel: [w295 w298] -> w197
          tunnel: w196 -> [_ w300]
          frame False {
          }
          frame True {
            n168 = Not(x=w297) -> (.not. x?=w296:bool)
            n169 = local write "set gas flow"(w296) -> ()
            n170 = local write "ramp down steps so far"(0 ("ramp down counter")) -> ()
            n171 = local write "ramp up steps so far"(0 ("ramp up counter")) -> ()
            n172 = local write "ramp down in progress"(FALSE ("ramp down in progress")) -> ()
            n173 = local write "ramp up in progress"(FALSE ("ramp up in progress")) -> ()
            n174 = call "ITC 503 -- set gas flow.vi"("error in"=w301, "Gas %"=w302, "ITC503 Address"=w300) -> ("error out"=w298:errorcluster)  [unwired: 7 in, 1 out]
          }
        }
        n175 = flat-sequence {
          tunnel: [w274] -> w270
          tunnel: w197 -> [w274]
          frame #0 {
            n176 = local read "ramp down in progress"() -> (w272:bool)
            n177 = local read "ramp up in progress"() -> (w273:bool)
            n178 = property on="ramp down steps so far" class="DigNum (strict)"("Visible"=w272) -> ()  [unwired: 2 in, 2 out]
            n179 = property on="ramp up steps so far" class="DigNum (strict)"("Visible"=w273) -> ()  [unwired: 2 in, 2 out]
            n180 = property on="ramp down in progress" class="Bool (strict)"("Visible"=w272) -> ()  [unwired: 2 in, 2 out]
            n181 = property on="ramp up in progress" class="Bool (strict)"("Visible"=w273) -> ()  [unwired: 2 in, 2 out]
          }
        }
      }
    }
    n182 = Unbundle By Name(w82) -> ("ITC temperature"=→"ITC Temperature":dbl, "ITC set temperature"=→"ITC Set T":dbl, "LTC temperature"=→"LTC Temperature":dbl, "heater"=→"heater voltage" →"heater":dbl, "gas flow"=→"Gas flow" →"gas flow %":dbl, "P"=→"P":dbl, "D"=→"D":dbl, "I"=→"I":dbl)  [unwired: 2 out]
    n183 = Unbundle By Name(w96) -> ("file path"=w122:path, "Save log?"=w121:bool, "every # of sec"=w120:i32)
    n184 = Quotient & Remainder(x=w89, y=w120) -> (x-y*floor(x/y)=w125:i32)  [unwired: 1 out]
    n185 = Equal To 0?(x=w125) -> (x = 0?=w124:bool)
    n186 = And(x=w124, y=w121) -> (x .and. y?=w123:bool)
    n187 = case shown="False" w123 {
      tunnel: w122 -> [_ w388]
      tunnel: [w384 w385] -> w117
      tunnel: w106 -> [w384 w386]
      tunnel: w82 -> [_ w387]
      frame False {
      }
      frame True {
        n188 = call "A - write log line.vi"("error in"=w386, "temperature boxes"=w387, "Basename"="Control_ITC_Log_" ("string"), "Base Path"=w388) -> ("error out"=w385:errorcluster, "saving log to"=w390:string)  [unwired: 6 in]
        n189 = local write "saving log to"(w390) -> ()
      }
    }
    n190 = Quotient & Remainder(x=w89, y=w88) -> (x-y*floor(x/y)=w90:u32)  [unwired: 1 out]
    n191 = Equal To 0?(x=w90) -> (x = 0?=w87:bool)
    n192 = case shown="True" w87 {
      tunnel: w117 -> [w169 w175]
      tunnel: w111 -> [_ w174]
      tunnel: [w169 w173] -> w110
      tunnel: w92 -> [w170 w172]
      tunnel: [w170 w171] -> w91
      frame False {
      }
      frame True {
        n193 = call "Control ITC Sweep -- aggregate state.vi"("error in"=w175, "more state"=w174, "more state -- aggregate in"=w172) -> ("error out"=w173:errorcluster, "more state -- aggregate out"=w171:T12)  [unwired: 7 in]
      }
    }
    n194 = local read "watch for sweep files in"() -> (w95:T8)
    n195 = Bundle By Name(cluster=w95, "file path"=w94) -> (w93:T8)
    n196 = Unbundle By Name(w93) -> ("Watch for sweep files?"=w130:bool)  [unwired: 1 out]
    n197 = local write "watch for sweep files in"(w93) -> ()
    n198 = local read "Overheat !!"() -> (w103:bool)
    n199 = disable-structure shown="Enabled" {
      disable-tunnel: w130 -> [w414 w419]
      disable-tunnel: [w413 w419] -> w129
      frame Disabled {
        # "check folder every ..."
        n200 = local read "seconds"() -> (w415:i32)
        n201 = Quotient & Remainder(x=w415, y=2) -> (x-y*floor(x/y)=w417:i32)  [unwired: 1 out]
        n202 = Equal To 0?(x=w417) -> (x = 0?=w416:bool)
        n203 = And(x=w414, y=w416) -> (x .and. y?=w413:bool)
      }
      frame Enabled {
      }
    }
    n204 = case shown="False" w129 {
      tunnel: w94 -> [_ w431]
      tunnel: w110 -> [w420 w421]
      tunnel: [w420 w421] -> w108
      frame False {
      }
      frame True {
        w430 = 60.0 ("y")
        # "hack"
        # "watch for new RUS file in sweep folder  and replace cursor every time sweep starts"
        # "date"
        n205 = Get Date/Time In Seconds() -> (seconds since 1Jan1904=w440:timestamp)
        n206 = Format Date/Time String(time format string (%c)="%m%d%y", seconds (now)=w440) -> (date/time string=w436:string)  [unwired: 1 in]
        n207 = Format Date/Time String(time format string (%c)="%B_%Y", seconds (now)=w440) -> (date/time string=w442:string)  [unwired: 1 in]
        n208 = Concatenate Strings(w442, "\\" ("time format string (%c)"), w436) -> (w443:string)
        n209 = Build Path(base path=w431, name or relative path=w443) -> (appended path=w433:path)
        n210 = Concatenate Strings("*" ("time format string (%c)"), w436, ".txt" ("time format string (%c)")) -> (w434:string)
        n211 = Path To String(path=w433) -> ()  [unwired: 1 out]
        n212 = call <vilib>:"Check if File or Folder Exists.vi"("path"=w433) -> ("file or folder exists?"=w423:bool, "dup path"=w432:path)  [unwired: 8 in, 1 out]
        n213 = local read "cursor position"() -> (w427:dbl)
        n214 = Multiply(x=w427, y=w430) -> (x*y=w428:dbl)
        n215 = Greater Or Equal To 0?(x=w427) -> (x >= 0?=w425:bool)
        n216 = Decrement(x=w428) -> (x-1=w429:dbl)
        n217 = Divide(x=w429, y=w430) -> (x/y=w426:dbl)
        n218 = And(x=w423, y=w425) -> (x .and. y?=w424:bool)
        n219 = Select(t=w426, s=w424, f=w427) -> (s? t:f=w422:dbl)
        n220 = local write "cursor position"(w422) -> ()
        n221 = property on="Plot: heater/gas" class="XYGraph (strict)"("Cursor.Cursor X"=w422) -> ()  [unwired: 2 in, 2 out]
        n222 = case shown="True" w423 {
          tunnel: w434 -> [_ w454]
          tunnel: w432 -> [_ w452]
          frame False {
            n223 = local read "watch for sweep files in"() -> (w446:T8)
            n224 = Bundle By Name(cluster=w446, "Watch for sweep files?"=FALSE) -> (w444:T8)
            n225 = local write "watch for sweep files in"(w444) -> ()
          }
          frame True {
            n226 = local read "sweep files in the folder"() -> (w449:i32)
            n227 = Less Than 0?(x=w449) -> (x < 0?=w448:bool)
            n228 = List Folder(path=w452, pattern=w454) -> (filenames=w453:string[])  [unwired: 2 in, 3 out]
            n229 = Array Size(array=w453) -> (size(s)=w451:i32)
            n230 = case shown="True" w448 {
              tunnel: w451 -> [_ w459]
              tunnel: [w458 w459] -> w450
              frame False {
                n231 = local read "sweep files in the folder"() -> (w458:i32)
              }
              frame True {
                n232 = local write "sweep files in the folder"(w459) -> ()
              }
            }
            n233 = Greater?(x=w451, y=w450) -> (0:w447:bool)
            n234 = case shown="True" w447 {
              tunnel: w447 -> [_ _]
              frame False {
              }
              frame True {
                n235 = local read "sweep files in the folder"() -> (w457:i32)
                n236 = local read "history length (min)"() -> (w455:dbl)
                n237 = Increment(x=w457) -> (x+1=w456:i32)
                n238 = local write "sweep files in the folder"(w456) -> ()
                n239 = local write "cursor position"(w455) -> ()
              }
            }
          }
        }
      }
    }
    n240 = case shown="False" w103 {
      tunnel: [w178 w194] -> w112
      tunnel: w108 -> [w177 w194]
      tunnel: w82 -> [w176 _]
      frame False {
        # "upload PID table"
        # "PID control"
        n241 = Unbundle By Name(w176) -> ("ITC503 Address"=w181:refnum<visa-resource-name>, "ITC temperature"=w180:dbl)
        n242 = local read "seconds"() -> (w179:i32)
        n243 = Quotient & Remainder(x=w179, y="PID update every") -> (x-y*floor(x/y)=w185:i32)  [unwired: 1 out]
        "cycles since PID update" <- w185
        n244 = Equal To 0?(x=w185) -> (x = 0?=w183:bool)
        n245 = And(x=w183, y="PID is") -> (x .and. y?=w182:bool)
        n246 = case shown="True" w182 {
          tunnel: "PID table" -> [_ w193]
          tunnel: [w188 w190] -> w178
          tunnel: w181 -> [_ w191]
          tunnel: w180 -> [_ w192]
          tunnel: w177 -> [w188 w189]
          frame False {
          }
          frame True {
            n247 = call "ITC 503 -- upload PID table.vi"("error in"=w189, "temperature"=w192, "PID table"=w193, "ITC503 Address"=w191) -> ("error out"=w190:errorcluster)  [unwired: 6 in, 1 out]
          }
        }
      }
      frame True {
      }
    }
    n248 = flat-sequence {
      tunnel: [w392] -> w109
      tunnel: w112 -> [w392]
      tunnel: w91 -> [w391]
      frame #0 {
        # "rate of heater change"
        # "Plot2"
        # "Plot 1"
        # "ITC -set"
        # "LTC - set"
        # "gas"
        # "heater"
        # "LTC temperature"
        # "ITC temperature"
        # "ITC set temperature"
        n249 = Unbundle By Name(w391) -> ("time(min)"=w400:dbl[], "T (ITC)  - T (ITC, set)"=w401:dbl[], "T (LTC)  - T (ITC, set)"=w402:dbl[], "heater"=w403:dbl[], "gas"=w404:dbl[], "heater slope"=w405:dbl[])
        n250 = Unbundle By Name(w391) -> ("time(min)"=w393:dbl[], "T (ITC, set)"=w396:dbl[], "T (ITC )"=w395:dbl[], "T (LTC)"=w394:dbl[])
        n251 = Bundle("time(min)"=w400, "T (ITC)  - T (ITC, set)"=w401) -> (w407:T15)  [unwired: 1 in]
        n252 = Bundle("time(min)"=w393, "T (ITC, set)"=w396) -> (w412:cluster{"time(min)":dbl[], "T (ITC, set)":dbl[]})  [unwired: 1 in]
        n253 = Bundle("time(min)"=w400, "T (LTC)  - T (ITC, set)"=w402) -> (w408:T16)  [unwired: 1 in]
        n254 = Bundle("time(min)"=w393, "T (ITC )"=w395) -> (w399:cluster{"time(min)":dbl[], "T (ITC )":dbl[]})  [unwired: 1 in]
        n255 = Bundle("time(min)"=w393, "T (LTC)"=w394) -> (w398:cluster{"time(min)":dbl[], "T (LTC)":dbl[]})  [unwired: 1 in]
        n256 = Bundle("time(min)"=w400, "heater"=w403) -> (w409:cluster{"time(min)":dbl[], "heater":dbl[]})  [unwired: 1 in]
        n257 = Bundle("time(min)"=w400, "gas"=w404) -> (w410:cluster{"time(min)":dbl[], "gas":dbl[]})  [unwired: 1 in]
        n258 = Bundle("time(min)"=w400, "heater slope"=w405) -> (w411:cluster{"time(min)":dbl[], "heater slope":dbl[]})  [unwired: 1 in]
        n259 = Build Array(w407, w408, w409, w410, w411) -> (→"Plot: heater/gas":T17)
        n260 = Build Array(w412, w399, w398) -> (→"Plot: temperature":cluster{"time(min)":dbl[], "T (LTC)":dbl[]}[])
      }
    }
    n261 = Unbundle By Name(w82) -> ("ITC503 Address"=w81:refnum<visa-resource-name>)
    n262 = disable-structure shown="Disabled" {
      disable-tunnel: [w356 w359] -> _
      disable-tunnel: w84 -> [w352 w359]
      frame Disabled {
        # "desperate attempt \nto keep ITC \nin local"
        n263 = local read "temperature boxes"() -> (w353:T6)
        n264 = Unbundle By Name(w353) -> ("ITC503 Address"=w354:refnum<visa-resource-name>)
        n265 = call "Oxford visa write read.vi"("error in (no error)"=w352, "write buffer"="C0" ("Command"), "VISA resource name"=w354) -> ("error out"=w355:errorcluster)  [unwired: 6 in, 2 out]
        n266 = call "Oxford visa write read.vi"("error in (no error)"=w355, "write buffer"="A1" ("Command"), "VISA resource name"=w354) -> ("error out"=w356:errorcluster)  [unwired: 6 in, 2 out]
      }
      frame Enabled {
      }
    }
    n267 = local read "seconds"() -> (w72:i32)
    n268 = Not(x="done") -> (.not. x?=w79:bool)
    n269 = Subtract(x=w72, y="to zero start (sec)") -> (x-y=w70:i32)
    n270 = Multiply(x="after (#min)", y=w73) -> (x*y=w85:dbl)
    n271 = Greater Or Equal?(x="to zero start (sec)", y=w75) -> (x >= y?=w74:bool)
    n272 = Greater?(x=w70, y=w85) -> (0:w76:bool)
    n273 = local write "to zero counter sec)"(w70) -> ()
    n274 = Compound Arithmetic op=AND(w79, w74, w76, "everything to zero") -> (w78:bool)
    n275 = case shown="True" w78 {
      selector: w78 -> [_ w146]
      tunnel: w84 -> [w143 w150]
      tunnel: [w143 w148] -> w83
      tunnel: w81 -> [_ w149]
      tunnel: FALSE -> [_ w145]
      tunnel: -1 -> [_ w144]
      frame False {
      }
      frame True {
        n276 = flat-sequence {
          tunnel: w150 -> [w159]
          tunnel: w149 -> [w158]
          tunnel: [w155] -> w147
          tunnel: [w168] -> w148
          tunnel: w147 -> [w168]
          frame #0 {
            w151 = "C0"  # write buffer
            w157 = 0.0  # Gas %
            # "stop sweep"
            # "Local locked"
            # "Heater V = 0"
            # "Heater Manual"
            # "Remote"
            n277 = for {
              tunnel: string[] ["C3", "A0", "S0", "O000"] -> [w164] mode=indexing
              shift-right: [w162] -> w153
              shift-left: w158 -> [w165]
              shift-right: [w161] -> w152
              shift-left: w159 -> [w163]
              n278 = call "Oxford visa write read.vi"("error in (no error)"=w163, "write buffer"=w164, "VISA resource name"=w165) -> ("error out"=w161:errorcluster, "VISA resource name out"=w162:refnum<visa-resource-name>)  [unwired: 6 in, 1 out]
            }
            n279 = call "ITC 503 -- set gas flow.vi"("error in"=w152, "Gas %"=w157, "ITC503 Address"=w153) -> ("error out"=w156:errorcluster, "ITC503 Address OUT"=w154:refnum<visa-resource-name>)  [unwired: 7 in]
            n280 = call "Oxford visa write read.vi"("error in (no error)"=w156, "write buffer"=w151, "VISA resource name"=w154) -> ("error out"=w155:errorcluster)  [unwired: 6 in, 2 out]
          }
          frame #1 {
            n281 = local write "Control Gas flow ?"(FALSE) -> ()
            n282 = local write "Stop RUS loop"(TRUE) -> ()
          }
        }
        n283 = local write "to zero start (sec)"(w144) -> ()
        n284 = local write "everything to zero"(w145) -> ()
        n285 = local write "done"(w146) -> ()
      }
    }
    "milliseconds per cycle" <- w142
    "seconds" <- w132
    "Global stop indicator" <- "event loop"
  }
  n286 = Unbundle By Name(w20) -> ("ITC503 Address"=w19:refnum<visa-resource-name>)
  n287 = property on="Uploading ..." class="Bool (strict)"("Visible"=w7) -> ()  [unwired: 2 in, 2 out]
  n288 = while {
    shift-right: [w462] -> w16
    shift-left: w17 -> [w463]
    tunnel: w11 -> [_]
    stop <- w465 stop-if-true
    n289 = local read "RUS loop"() -> (w464:bool)
    n290 = case shown="True" w464 {
      tunnel: [w468 w472] -> w461
      tunnel: w463 -> [w468 w471]
      frame False {
      }
      frame True {
        n291 = while {
          tunnel: "at end of every sweep" -> [w508]
          shift-right: [w494] -> w472
          shift-left: w471 -> [w475]
          tunnel: "wait time between sweeps (min)" -> [w497]
          stop <- w485 continue-if-true
          w480 = TRUE  # Bypass Errors
          (unwired) FALSE ("frequency  format")
          (unwired) TRUE ("set amplitude to zero \nat end of every sweep")
          n292 = local read "temperature boxes"() -> (w473:T6)
          n293 = Equal To 0?(x=w497) -> (x = 0?=w499:bool)
          n294 = Select(t=0.0001, s=w499, f=w497) -> (s? t:f=w498:dbl)
          n295 = Unbundle By Name(w473) -> ("nonzero temperature"=w474:dbl)
          n296 = Multiply(x=w498, y=60000.0) -> (x*y=w500:dbl)
          n297 = Wait (ms)(milliseconds to wait=w500) -> ()  [unwired: 1 out]
          n298 = call "file name prefix.vi"("Fast sweep settings"="Fast sweep settings", "temperature"=w474) -> ("minutes/sweep"=→"minutes/sweep":dbl, "kHz/second"=→"kHz/second":dbl, "file name prefix"=w489:string)  [unwired: 7 in]
          n299 = Bundle By Name(cluster="Save data settings", "File Prefix"=w489) -> (w493:T4)
          n300 = call "RUS Sweep -- build content of txt file.vi"("temperature boxes"=w473, "error in"=w475, "Save data settings"=w493) -> ("error out"=w503:errorcluster, "Save data settings out"=w492:T4)  [unwired: 7 in]
          n301 = Unbundle By Name(w492) -> ("Data Root Path"=w484:path, "File Prefix"=w491:string)
          n302 = call "App - RUS scan V0.vi"("Bypass error dialog"="Bypass error dialog", "Divide something by something for Albert"="save frequency in", "Zero amplitude at the end"=w508, "Save data settings"=w492, "error in (no error)"=w503, "Fast swep settings"="Fast sweep settings", "Lock-in DAQ settings"="Lock-in DAQ settings") -> ("error out"=w477:errorcluster, "Actual file path"=w502:path)  [unwired: 2 in, 1 out]
          n303 = Build Path(base path=w484, name or relative path="ErrorLog.txt") -> (appended path=w482:path)
          n304 = call "RUS Sweep -- write line to Temperatures file.vi"("error in"=w477, "Folder Path"=w502, "LTC Temperature"=w474) -> ("error out"=w479:errorcluster)  [unwired: 8 in]
          n305 = call "BypassAndLogErrors.vi"("Bypass Errors"=w480, "error in (no error)"=w479, "Log File Path"=w482) -> ("error out"=w478:errorcluster)  [unwired: 8 in]
          n306 = call "RUS Sweep -- write line to log file.vi"("temperature boxes"=w473, "base path"=w484, "error in (no error)"=w478, "current sweep file name"=w491, "base name"="Stability_") -> ("error out"=w494:errorcluster, "writing to"=→"writing log to":string, "log line"=→"log line":string)  [unwired: 4 in]
          n307 = Not(x="Stop RUS loop") -> (.not. x?=w485:bool)
        }
      }
    }
    n308 = Wait (ms)(milliseconds to wait=1500.0 ("y")) -> ()  [unwired: 1 out]
    n309 = local read "Global stop indicator"() -> (w465:bool)
    n310 = flat-sequence {
      tunnel: [w467] -> w462
      tunnel: w461 -> [w467]
      frame #0 {
        w466 = FALSE ("GO!")
        n311 = local write "Stop RUS loop"(w466) -> ()
        n312 = local write "RUS loop"(w466) -> ()
      }
    }
  }
  n313 = while {
    shift-right: [w518] -> w18
    shift-left: w17 -> [w520]
    tunnel: w19 -> [w519]
    tunnel: w7 -> [_]
    tunnel: w15 -> [_]
    tunnel: w14 -> [_]
    tunnel: "watch for sweep files in" -> [_]
    tunnel: [w513] -> w10
    tunnel: w8 -> [_]
    stop <- w513 stop-if-true
    w511 = T18."parse"  # action
    n314 = Wait (ms)(milliseconds to wait=u32 300 ("milliseconds per cycle")) -> ()  [unwired: 1 out]
    n315 = control-ref of="ITC panel"() -> (w509:refnum<vi>)
    n316 = event shown="[10] \"ITC panel.start/stop sweep\": Value Change" {
      selector: _ -> [_ _ _ _ _ _ _ _ _ _ _]
      dyn-events: _ -> [_ _ _ _ _ _ _ _ _ _ _]
      timeout: 100 -> [_ _ _ _ _ _ _ _ _ _ _]
      tunnel: [w523 _ _ _ _ _ _ _ _ _ _] -> w515
      tunnel: [_ _ "upload new sweep table" _ _ _ _ _ _ _ _] -> _
      tunnel: w520 -> [w522 _ w538 w562 w565 w583 _ w605 w613 w628 w644]
      tunnel: [w522 _ w535 w560 _ w580 _ _ w611 w624 w645] -> w518
      tunnel: w519 -> [_ _ w549 _ _ w582 _ w606 w612 w627 w643]
      tunnel: [_ _ FALSE _ _ _ _ _ _ _ _] -> _
      tunnel: [_ _ _ _ _ "Read Sweep Table in the box" _ _ _ _ _] -> _
      tunnel: [_ _ _ _ _ _ _ "set temperature to" _ _ _] -> _
      tunnel: [_ _ _ _ _ _ _ w596 _ _ _] -> _
      tunnel: [_ _ _ _ "upload new sweep sequence" _ _ _ _ _ _] -> _
      tunnel: [_ _ _ _ w565 _ _ _ _ _ _] -> _
      tunnel: [_ _ _ w559 _ _ _ _ _ _ _] -> _
      tunnel: TRUE -> [_ _ w539 _ _ _ _ _ _ _ _]
      event Timeout {
        n317 = event-data() -> ()  [unwired: 1 in, 2 out]
        n318 = local read "Global stop indicator"() -> (w523:bool)
      }
      event "everything to zero": Value Change {
        n319 = event-data() -> ("NewVal"=w528:bool)  [unwired: 1 in, 4 out]
        n320 = local read "seconds"() -> (w527:i32)
        n321 = case shown="False" w528 {
          tunnel: w527 -> [_ w533]
          tunnel: FALSE -> [w529 w532]
          tunnel: TRUE -> [_ w531]
          tunnel: -1 -> [w530 _]
          frame False {
            n322 = local write "done"(w529) -> ()
            n323 = local write "to zero start (sec)"(w530) -> ()
            n324 = property on="to zero counter sec)" class="DigNum (strict)"("Visible"=w529) -> ()  [unwired: 2 in, 2 out]
          }
          frame True {
            n325 = local write "to zero start (sec)"(w533) -> ()
            n326 = local write "done"(w532) -> ()
            n327 = property on="to zero counter sec)" class="DigNum (strict)"("Visible"=w531) -> ()  [unwired: 2 in, 2 out]
          }
        }
      }
      event "upload new sweep table": Value Change {
        w534 = FALSE
        n328 = event-data() -> ()  [unwired: 1 in, 1 out]
        n329 = local read "Save data settings"() -> (w543:T4)
        n330 = local write "Uploading ..."(w539) -> ()
        n331 = property on="Uploading ..." class="Bool (strict)"(error in=w538, "Visible"=w539) -> (error out=w537:errorcluster)  [unwired: 1 in, 1 out]
        n332 = Unbundle By Name("Save sweep table") -> ("Save sweep table?"=w540:bool)
        n333 = Unbundle By Name(w543) -> ("Data Root Path"=w542:path)
        n334 = call "ITC 503 -- upload sweep table.vi"("error in"=w537, "Start set point"="start \nset temperature", "Sweep Table"="New Sweep Table", "ITC503 Address"=w549) -> ("error out"=w548:errorcluster)  [unwired: 6 in, 1 out]
        n335 = case shown="True" w540 {
          tunnel: w542 -> [_ w558]
          tunnel: w548 -> [w551 w556]
          tunnel: [w551 w555] -> w536
          tunnel: "start \nset temperature" -> [_ w553]
          tunnel: "New Sweep Table" -> [_ w552]
          frame False {
          }
          frame True {
            n336 = call "ITC 503 -- save sweep table.vi"("Set Temperature"=w553, "Sweep Table"=w552, "error in"=w556, "Base Path"=w558, "Base name"="SweepTable_" ("string")) -> ("error out"=w555:errorcluster, "saving sweep table to"=w557:string)  [unwired: 5 in]
            n337 = local write "saving sweep table to"(w557) -> ()
          }
        }
        n338 = Bundle By Name(cluster="Save sweep table", "file path"=w542) -> (w544:T9)
        n339 = local write "Save sweep table"(w544) -> ()
        n340 = local write "Uploading ..."(w534) -> ()
        n341 = property on="Uploading ..." class="Bool (strict)"(error in=w536, "Visible"=w534) -> (error out=w535:errorcluster)  [unwired: 1 in, 1 out]
      }
      event "show plot pallets": Value Change {
        n342 = event-data() -> ("NewVal"=w559:bool)  [unwired: 1 in]
        n343 = control-ref of="Plot: heater/gas"() -> (w563:refnum<vi>)
        n344 = control-ref of="Plot: temperature"() -> (w564:refnum<vi>)
        n345 = property on="Property Node" class="XYGraph (strict)"(reference=w564, error in=w562, "ScaleLegendVis"=w559, "Palette Visible"=w559, "Legend Visible"=w559) -> (error out=w561:errorcluster)  [unwired: 1 out]
        n346 = property on="Property Node" class="XYGraph (strict)"(reference=w563, error in=w561, "ScaleLegendVis"=w559, "Palette Visible"=w559, "Legend Visible"=w559) -> (error out=w560:errorcluster)  [unwired: 1 out]
      }
      event "upload new sweep sequence": Value Change {
        n347 = event-data() -> ()  [unwired: 1 in, 5 out]
      }
      event "Read Sweep Table in the box": Value Change {
        # "read sweep table"
        n348 = event-data() -> ()  [unwired: 1 in, 5 out]
        n349 = call "ITC 503 -- read sweep table.vi"("error in"=w583, "ITC503 Address"=w582) -> ("error out"=w581:errorcluster, "Sweep Table"=w573:dbl[][], "ITC503 Address OUT"=w579:refnum<visa-resource-name>)  [unwired: 7 in]
        "Sweep Table" <- w573
        n350 = call "Oxford Read Channel.vi"("error in (no error)"=w581, "Channel #"=0 ("Sensor #"), "VISA resource name"=w579) -> ("error out"=w580:errorcluster, "Data"=w572:dbl)  [unwired: 5 in, 2 out]
        "current set \ntemperature" <- w572
        n351 = Array Size(array=w573) -> (size(s)=w577:i32[])
        n352 = Index Array(array=w577, index=0) -> (element=w570:i32)
        n353 = Initialize Array(0.0 ("element"), w570) -> (w574:dbl[])
        n354 = for {
          N: w570 -> [_]
          shift-right: [w592] -> w571
          shift-left: w574 -> [w594]
          tunnel: w573 -> [w590] mode=indexing
          shift-right: [w586] -> _
          shift-left: w572 -> [w585]
          i -> [w593]
          n355 = Index Array(array=w590, index=0) -> (element=w586:dbl)
          n356 = Subtract(x=w586, y=w585) -> (x-y=w589:dbl)
          n357 = Index Array(array=w590, index=1) -> (element=w588:dbl)
          n358 = Divide(x=w589, y=w588) -> (x/y=w587:dbl)
          n359 = Replace Array Subset(array=w594, new element=w587, index=w593) -> (w592:dbl[])
        }
        n360 = Reshape Array(w571, w570, 1 ("dimension size")) -> (w567:dbl[][])
        "Sweep Rates ,\nK/min" <- w567
        n361 = Reciprocal(x=w567) -> (1/x=→"Sweep Rates , \nmin/K":dbl[][])
      }
      event Key Down {
        n362 = event-data() -> ()  [unwired: 1 in, 2 out]
      }
      event "set temperature to": Value Change {
        n363 = event-data() -> ()  [unwired: 1 in, 5 out]
        n364 = call "Oxford visa write read.vi"("error in (no error)"=w605, "write buffer"="C3" ("Command"), "VISA resource name"=w606) -> ("error out"=w609:errorcluster, "VISA resource name out"=w608:refnum<visa-resource-name>)  [unwired: 6 in, 1 out]
        n365 = Number To Fractional String(number="set temperature to", precision (6)=i16 1) -> (F-format string=w601:string)  [unwired: 2 in]
        n366 = Concatenate Strings("T" ("Command"), w601) -> (w599:string)
        n367 = call "Oxford visa write read.vi"("error in (no error)"=w609, "write buffer"=w599, "VISA resource name"=w608) -> ("error out"=w597:errorcluster, "VISA resource name out"=w598:refnum<visa-resource-name>)  [unwired: 6 in, 1 out]
        n368 = call "Oxford visa write read.vi"("error in (no error)"=w597, "write buffer"="C2" ("Command"), "VISA resource name"=w598) -> ("error out"=w596:errorcluster)  [unwired: 6 in, 2 out]
      }
      event Value Change {
        n369 = event-data() -> ()  [unwired: 1 in, 5 out]
        n370 = call "Oxford visa write read.vi"("error in (no error)"=w613, "write buffer"="C3" ("Command"), "VISA resource name"=w612) -> ("error out"=w615:errorcluster, "VISA resource name out"=w618:refnum<visa-resource-name>)  [unwired: 6 in, 1 out]
        n371 = call "Oxford visa write read.vi"("error in (no error)"=w615, "write buffer"="A0" ("Command"), "VISA resource name"=w618) -> ("error out"=w614:errorcluster, "VISA resource name out"=w617:refnum<visa-resource-name>)  [unwired: 6 in, 1 out]
        n372 = call "Oxford visa write read.vi"("error in (no error)"=w614, "write buffer"="O000" ("Command"), "VISA resource name"=w617) -> ("error out"=w622:errorcluster, "VISA resource name out"=w621:refnum<visa-resource-name>)  [unwired: 6 in, 1 out]
        n373 = call "Oxford visa write read.vi"("error in (no error)"=w622, "write buffer"="C2" ("Command"), "VISA resource name"=w621) -> ("error out"=w611:errorcluster)  [unwired: 6 in, 2 out]
      }
      event Value Change {
        n374 = event-data() -> ()  [unwired: 1 in, 5 out]
        n375 = call "Oxford visa write read.vi"("error in (no error)"=w628, "write buffer"="C3" ("Command"), "VISA resource name"=w627) -> ("error out"=w633:errorcluster, "VISA resource name out"=w631:refnum<visa-resource-name>)  [unwired: 6 in, 1 out]
        n376 = call "Oxford visa write read.vi"("error in (no error)"=w633, "write buffer"="A1" ("Command"), "VISA resource name"=w631) -> ("error out"=w625:errorcluster, "VISA resource name out"=w626:refnum<visa-resource-name>)  [unwired: 6 in, 1 out]
        n377 = call "Oxford visa write read.vi"("error in (no error)"=w625, "write buffer"="C2" ("Command"), "VISA resource name"=w626) -> ("error out"=w624:errorcluster)  [unwired: 6 in, 2 out]
      }
      event Value Change {
        n378 = event-data() -> ()  [unwired: 1 in, 5 out]
        n379 = local read "ITC panel"() -> (w634:T7)
        n380 = Unbundle By Name(w634) -> ("in sweep"=w635:bool)
        n381 = call "Oxford visa write read.vi"("error in (no error)"=w644, "write buffer"="C3" ("Command"), "VISA resource name"=w643) -> ("error out"=w638:errorcluster, "VISA resource name out"=w637:refnum<visa-resource-name>)  [unwired: 6 in, 1 out]
        n382 = case shown="True" w635 {
          tunnel: ["S1" ("write buffer") "S0" ("write buffer")] -> w642
          frame False {
            # "start sweep ..."
          }
          frame True {
            # "stop sweep ..."
          }
        }
        n383 = call "Oxford visa write read.vi"("error in (no error)"=w638, "write buffer"=w642, "VISA resource name"=w637) -> ("error out"=w641:errorcluster, "VISA resource name out"=w639:refnum<visa-resource-name>)  [unwired: 6 in, 1 out]
        n384 = call "Oxford visa write read.vi"("error in (no error)"=w641, "write buffer"="C2" ("Command"), "VISA resource name"=w639) -> ("error out"=w645:errorcluster)  [unwired: 6 in, 2 out]
      }
    }
    n385 = local read "temperature boxes"() -> (w512:T6)
    n386 = call "ITC panel control.vi"("temperature boxes"=w512, "action"=w511, "ITC panel IN"=w509) -> ()  [unwired: 8 in, 1 out]
    n387 = local read "Overheat !!"() -> (w514:bool)
    n388 = Unbundle By Name(w518) -> ("status"=w516:bool)
    n389 = Compound Arithmetic op=OR(w516, w515, w514) -> (w513:bool)
  }
  n390 = flat-sequence {
    tunnel: w10 -> [w649]
    frame #0 {
      n391 = for {
        tunnel: w649 -> [w657]
        tunnel: i32[] [3, 4, 5, 6] -> [w653] mode=indexing
        # "pid contro page"
        n392 = property on="everything" class="TabCtl (strict)"() -> ("Pages"=w659:refnum<vi>[])  [unwired: 2 in, 2 out]
        n393 = Select(t=T14."Page Disabled & Grayed" ("Page Enabled State"), s=w657, f=T14."Page Enabled" ("Page Enabled State")) -> (s? t:f=w654:T14)
        n394 = Index Array(array=w659, index=w653) -> (element=w658:refnum<vi>)
        n395 = property on="Property Node" class="Page"(reference=w658, "PageEnb"=w654) -> ()  [unwired: 1 in, 2 out]
      }
      n396 = Select(t=T13."Disabled and Grayed Out" ("Disabled"), s=w649, f=T13."Enabled" ("Disabled")) -> (s? t:f=w650:T13)
      n397 = property on="TAB: gas flow control" class="TabCtl (strict)"("DisabledEnum"=w650) -> ()  [unwired: 2 in, 2 out]
      n398 = property on="Tab: ITC controls" class="TabCtl (strict)"("DisabledEnum"=w650) -> ()  [unwired: 2 in, 2 out]
    }
  }
  n399 = disable-structure shown="Disabled" {
    frame Disabled {
      n400 = flat-sequence {
        tunnel: _ -> [w701]
        tunnel: _ -> [w693]
        tunnel: _ -> [w675]
        tunnel: [w673] -> w660
        tunnel: _ -> [w671]
        tunnel: [w661] -> _
        tunnel: _ -> [w661]
        frame #0 {
          # "LTC minus ITC_set"
          # "ITC minus ITC_set"
          n401 = local read item#-1() -> (w662)
          n402 = Unbundle By Name(w662) -> ("time(min)"=w690, "T (ITC )"=w688, "T (ITC, set)"=w686, "T (LTC)"=w683, "heater"=w682, "gas"=w679, "T (ITC)  - T (ITC, set)"=w669, "T (LTC)  - T (ITC, set)"=w664, "heater slope"=w665, "LTC slope"=w666, "hetaer running average"=w667, "T (LTC) running average"=w668)
          n403 = local read item#-1() -> (w691)
          n404 = local read item#-1() -> (w692)
          n405 = Build Array (concatenate)(w690, w692) -> (w689:void[])
          n406 = Unbundle By Name(w691) -> ("ITC temperature"=w697, "ITC set temperature"=w700, "LTC temperature"=w696, "heater"=w699, "gas"=w698)
          n407 = Subtract(x=w697, y=w701) -> (x-y=w695:dbl)
          n408 = Subtract(x=w696, y=w701) -> (x-y=w694:dbl)
          n409 = Build Array (concatenate)(w688, w697) -> (w687:void[])
          n410 = Build Array (concatenate)(w686, w700) -> (w685:void[])
          n411 = Build Array (concatenate)(w683, w696) -> (w684:void[])
          n412 = Build Array (concatenate)(w682, w699) -> (w681:void[])
          n413 = Build Array (concatenate)(w668, w671) -> (w670:void[])
          n414 = Build Array (concatenate)(w679, w698) -> (w680:void[])
          n415 = Build Array (concatenate)(w667, w673) -> (w672:void[])
          n416 = Build Array (concatenate)(w669, w695) -> (w678:dbl[])
          n417 = Build Array (concatenate)(w664, w694) -> (w677:dbl[])
          n418 = Build Array (concatenate)(w666, w675) -> (w674:void[])
          n419 = Build Array (concatenate)(w665, w693) -> (w676:void[])
          n420 = Bundle By Name(cluster=w662, "time(min)"=w689, "T (ITC )"=w687, "T (ITC, set)"=w685, "T (LTC)"=w684, "heater"=w681, "gas"=w680, "T (ITC)  - T (ITC, set)"=w678, "T (LTC)  - T (ITC, set)"=w677, "heater slope"=w676, "LTC slope"=w674, "hetaer running average"=w672, "T (LTC) running average"=w670) -> (w663:cluster{})
          n421 = local write item#-1(w663) -> ()
        }
      }
    }
    frame Enabled {
    }
  }
  n422 = flat-sequence {
    tunnel: [w702] -> w1
    frame #0 {
      w702 = FALSE  # everything to zero
      # "init for \"everything to zero\""
      n423 = property on="to zero counter sec)" class="DigNum (strict)"("Visible"=w702) -> ()  [unwired: 2 in, 2 out]
      n424 = local write "everything to zero"(w702) -> ()
      n425 = local write "done"(w702) -> ()
      n426 = local write "to zero counter sec)"(0) -> ()
      n427 = local write "to zero start (sec)"(-1) -> ()
    }
  }
  n428 = Merge Errors(w16, w23, w18) -> (→"error out":errorcluster)
  "Uploading ..." <- w7
  "sweep files in the folder" <- w15
  "history length (min)" <- w29
  "cursor position" <- w14
  "saving log to" <- ""
  "saving sweep table to" <- "" ("saving sweep table to")
  "Overheat !!" <- w12
